vi "FindPOSCheckPercentDiff (SubVI).vi"(0 "x":sgl, 1 "y":sgl, 2 "true x":sgl, 3 "true y":sgl, 4 "variation tolerance":sgl) -> (7 "pass x coordinate":bool, 8 "pass y coordinate":bool, 9 "delta X":sgl, 10 "delta Y":sgl)   [LabVIEW 2016]
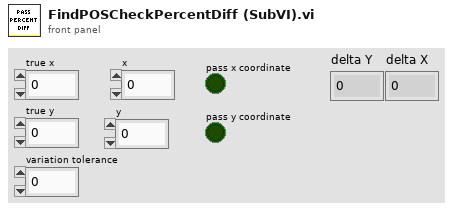
[diagram p1: front panel]
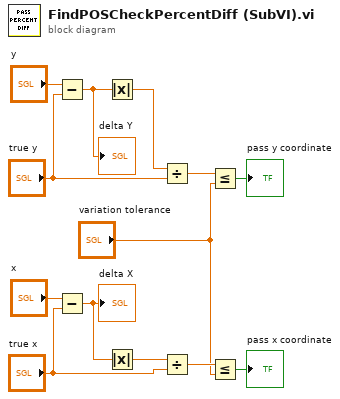
[diagram p0: block diagram]
diagram:
  n1 = Subtract(x="y", y="true y") -> (x-y=w11:sgl)
  "delta Y" <- w11
  n2 = Subtract(x="x", y="true x") -> (x-y=w5:sgl)
  "delta X" <- w5
  n3 = Absolute Value(x=w11) -> (abs(x)=w10:sgl)
  n4 = Absolute Value(x=w5) -> (abs(x)=w6:sgl)
  n5 = Divide(x=w10, y="true y") -> (x/y=w9:sgl)
  n6 = Divide(x=w6, y="true x") -> (x/y=w7:sgl)
  n7 = Less Or Equal?(x=w9, y="variation tolerance") -> (x <= y?=→"pass y coordinate":bool)
  n8 = Less Or Equal?(x=w7, y="variation tolerance") -> (x <= y?=→"pass x coordinate":bool)
